vi "Global_CMD.vi"() -> ()   [LabVIEW 2017, in "System_Status.lvlib"]
uses:
  System_Status.lvlib
  CLUSTER_System_CMD.ctl
panel:
  in  "System_Status_CMD":T1
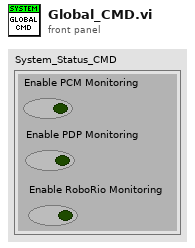
[diagram p1: front panel]
types:
  T1 = typedef "System_Status.lvlib/CLUSTER_System_CMD.ctl" = cluster{"Enable PCM Monitoring":bool, "Enable PDP Monitoring":bool, "Enable RoboRio Monitoring":bool}
diagram:
